vi "BooleanToStringSub.vi"(11 "Relay Switch":bool) -> (3 "Numeric":i32)   [LabVIEW 2026]
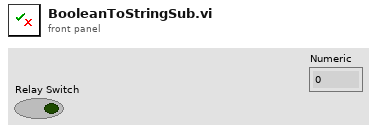
[diagram p1: front panel]
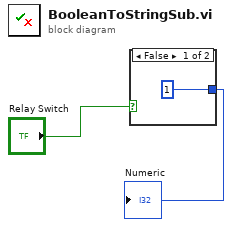
[diagram p0: block diagram]
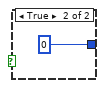
[diagram p2: hidden frame]
diagram:
  n1 = case shown="False" "Relay Switch" {
    tunnel: [1 0] -> w1
    frame False {
    }
    frame True {
    }
  }
  "Numeric" <- w1
